vi "ALTS-2015 LV2GBL Control Reference.vi"(6 "LV2 Options":T2, 8 "error in":errorcluster, 11 "Control Reference_In":T1) -> (0 "error out":errorcluster, 3 "Control Reference_Out":T1)   [LabVIEW 2013]
uses:
  Controls/ALTS-2015 Control Reference LV2 Options.ctl
  Controls/ALTS-2015 Control Reference.ctl
  Controls/ALTS-2015 Station Details.ctl
  Controls/ALTS-2015 Status Ring Indicator.ctl
  Controls/ALTS-2015 Robot Actions.ctl
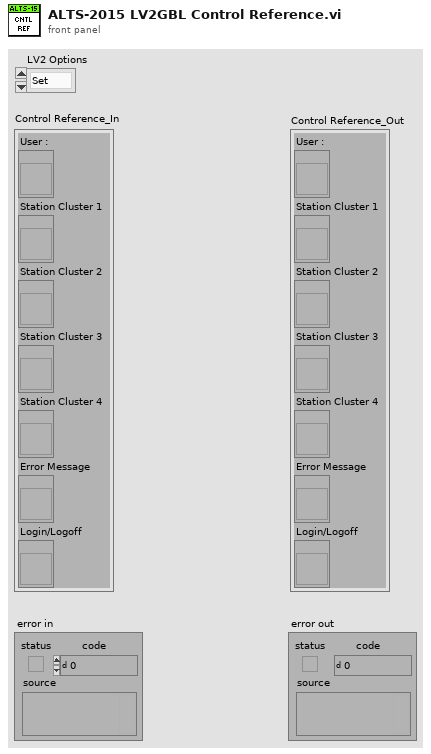
[diagram p1: front panel]
types:
  T1 = typedef "ALTS-2015 Control Reference.ctl" = cluster{"User :":refnum<vi>, "Station Cluster 1":refnum<vi>, "Station Cluster 2":refnum<vi>, "Station Cluster 3":refnum<vi>, "Station Cluster 4":refnum<vi>, "Error Message":refnum<vi>, "Login/Logoff":refnum<vi>}
  T2 = typedef "ALTS-2015 Control Reference LV2 Options.ctl" = enum16{"Set", "Get"}
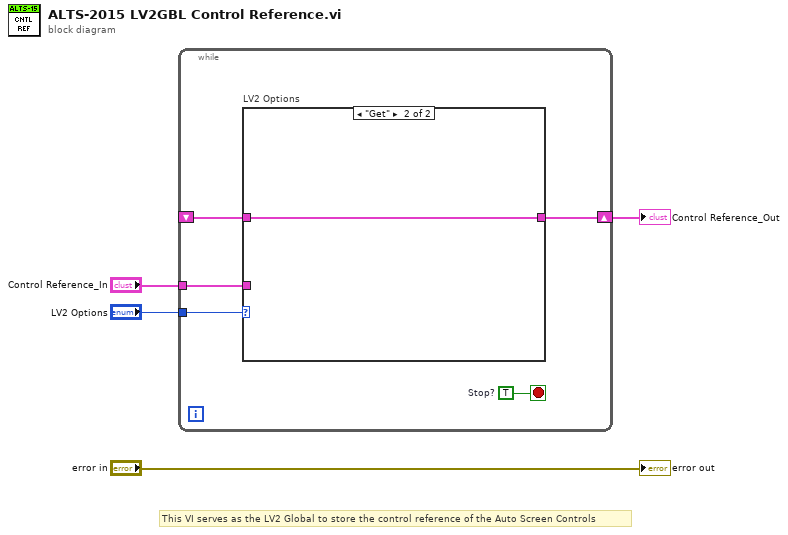
[diagram p0: block diagram]
diagram:
  # "This VI serves as the LV2 Global to store the control reference of the Auto Screen Controls"
  n1 = while {
    tunnel: "LV2 Options" -> [w9]
    shift-right: [w7] -> w2
    shift-left: _ -> [w6]
    tunnel: "Control Reference_In" -> [w8]
    stop <- w5 stop-if-true
    w5 = TRUE  # Stop?
    n2 = case "LV2 Options" shown="\"Get\"" w9 {
      tunnel: w8 -> [w10 _]
      tunnel: [w10 w11] -> w7
      tunnel: w6 -> [_ w11]
      frame "Set" {
      }
      frame "Get" {
      }
    }
  }
  "Control Reference_Out" <- w2
  "error out" <- "error in"
